vi "Acquire.vi"(8 "error in (no error)":errorcluster, 9 "Data Queue":refnum<queue>, 10 "Data Notifier":refnum<notifier>, 11 "Hardware Resources in":T1={"AI"={"task name"="", "task_ref"="", "physical channels"="Dev1/ai0:7", "channels config"={"input terminal configuration"=0, "minimum value"=-5.0, "maximum value"=5.0}, "rate"=1000.0}, "conversions"={"ai0"={"a"=0.0, "b"=0.0}, "ai1"={"a"=0.0, "b"=0.0}, "ai2"={"a"=0.0, "b"=0.0}, "ai3"={"a"=0.0, "b"=0.0}, "ai4"={"a"=0.0, "b"=0.0}}, "compteur 0"={"task name"="CTR", "task_ref"="", "ctr"="Dev1/ctr0:3", "coeff"=4000.0}, "compteur 1"={"task name"="CTR1", "task_ref"="", "ctr"="Dev1/ctr1", "coeff"=4000.0}, "compteur 2"={"task name"="CTR2", "task_ref"="", "ctr"="Dev1/ctr2", "coeff"=4000.0}, "compteur 3"={"task name"="CTR3", "task_ref"="", "ctr"="Dev1/ctr3", "coeff"=4000.0}} {"compteur 3"."coeff" format="%0.2f"; "compteur 2"."coeff" format="%0.2f"; "compteur 1"."coeff" format="%0.2f"; "compteur 0"."coeff" format="%0.2f"; "AI"."rate" format="%0.2f"; "AI"."channels config"."input terminal configuration" items=["Default"=-1, "RSE"=10083, "NRSE"=10078, "Differential"=10106, "Pseudodifferential"=12529]}) -> (0 "error out":errorcluster, 3 "Hardware Resources out":T1={"AI"={"task name"="", "task_ref"="", "physical channels"="Dev1/ai0:7", "channels config"={"input terminal configuration"=0, "minimum value"=-5.0, "maximum value"=5.0}, "rate"=1000.0}, "conversions"={"ai0"={"a"=0.0, "b"=0.0}, "ai1"={"a"=0.0, "b"=0.0}, "ai2"={"a"=0.0, "b"=0.0}, "ai3"={"a"=0.0, "b"=0.0}, "ai4"={"a"=0.0, "b"=0.0}}, "compteur 0"={"task name"="CTR", "task_ref"="", "ctr"="Dev1/ctr0:3", "coeff"=4000.0}, "compteur 1"={"task name"="CTR1", "task_ref"="", "ctr"="Dev1/ctr1", "coeff"=4000.0}, "compteur 2"={"task name"="CTR2", "task_ref"="", "ctr"="Dev1/ctr2", "coeff"=4000.0}, "compteur 3"={"task name"="CTR3", "task_ref"="", "ctr"="Dev1/ctr3", "coeff"=4000.0}} {"compteur 3"."coeff" format="%0.2f"; "compteur 2"."coeff" format="%0.2f"; "compteur 1"."coeff" format="%0.2f"; "compteur 0"."coeff" format="%0.2f"; "AI"."rate" format="%0.2f"; "AI"."channels config"."input terminal configuration" items=["Default"=-1, "RSE"=10083, "NRSE"=10078, "Differential"=10106, "Pseudodifferential"=12529]})   [LabVIEW 2014, in "PLS Acquisition.lvlib"]
doc: "Perform the acquisition. Replace the contents of this diagram with calls to acquisition hardware."
uses:
  PLS Acquisition.lvlib
  Hardware Configuration.ctl
  Settings/conversion.ctl
  <vilib>/DAQmx/read.llb/DAQmx Read (Counter DBL 1Chan 1Samp).vi
  <vilib>/DAQmx/read.llb/DAQmx Read (Analog 1D Wfm NChan NSamp).vi
  <vilib>/DAQmx/miscellaneous.llb/DAQmx Fill In Error Info.vi
  GLB_compteurs.vi
  GLB_Fsave.vi
  Settings/PLS Settings.lvlib
panel:
  out "d4":i32=10
  out "d3":i32=10
  out "d2":i32=10
  out "d1":i32=10
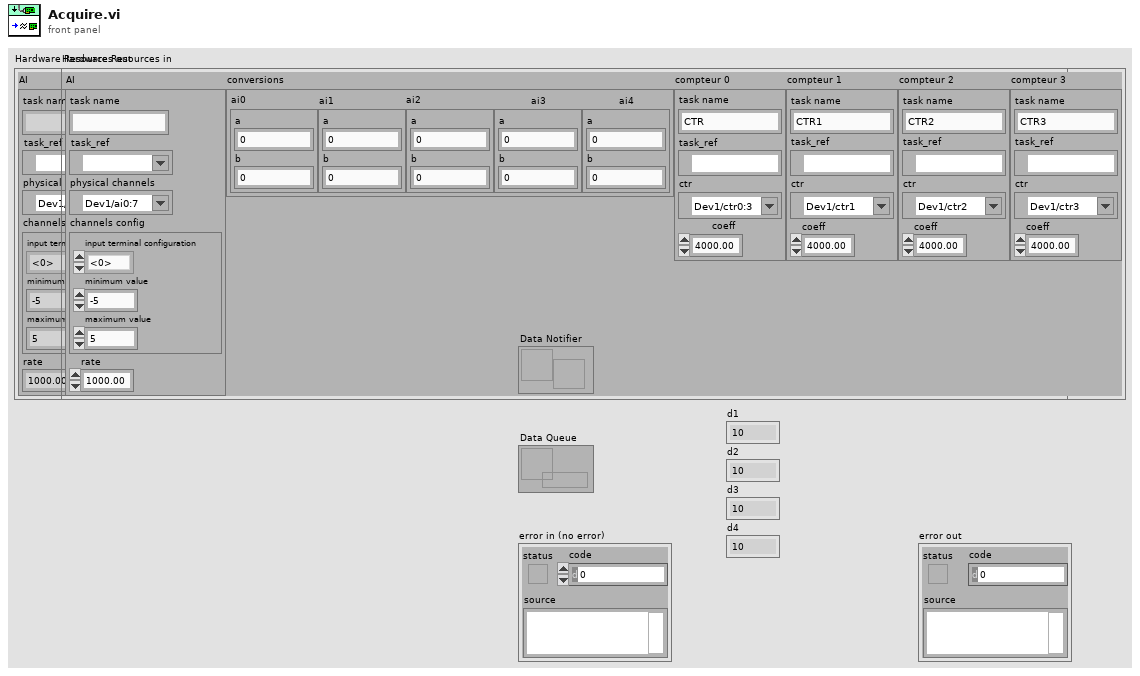
[diagram p1: front panel]
types:
  T1 = typedef "PLS Acquisition.lvlib/Hardware Configuration.ctl" = cluster{"AI":cluster{"task name":string, "task_ref":refnum<k21>, "physical channels":tag, "channels config":cluster{"input terminal configuration":i32, "minimum value":dbl, "maximum value":dbl}, "rate":dbl}, "conversions":cluster{"ai0":T2, "ai1":T2, "ai2":T2, "ai3":T2, "ai4":T2}, "compteur 0":cluster{"task name":string, "task_ref":refnum<k21>, "ctr":tag, "coeff":dbl}, "compteur 1":cluster{"task name":string, "task_ref":refnum<k21>, "ctr":tag, "coeff":dbl}, "compteur 2":cluster{"task name":string, "task_ref":refnum<k21>, "ctr":tag, "coeff":dbl}, "compteur 3":cluster{"task name":string, "task_ref":refnum<k21>, "ctr":tag, "coeff":dbl}}
  T2 = typedef "PLS Settings.lvlib/conversion.ctl" = cluster{"a":dbl, "b":dbl}
  T3 = cluster{"ai0":T2, "ai1":T2, "ai2":T2, "ai3":T2, "ai4":T2}
  T4 = cluster{"task name":string, "task_ref":refnum<k21>, "ctr":tag, "coeff":dbl}
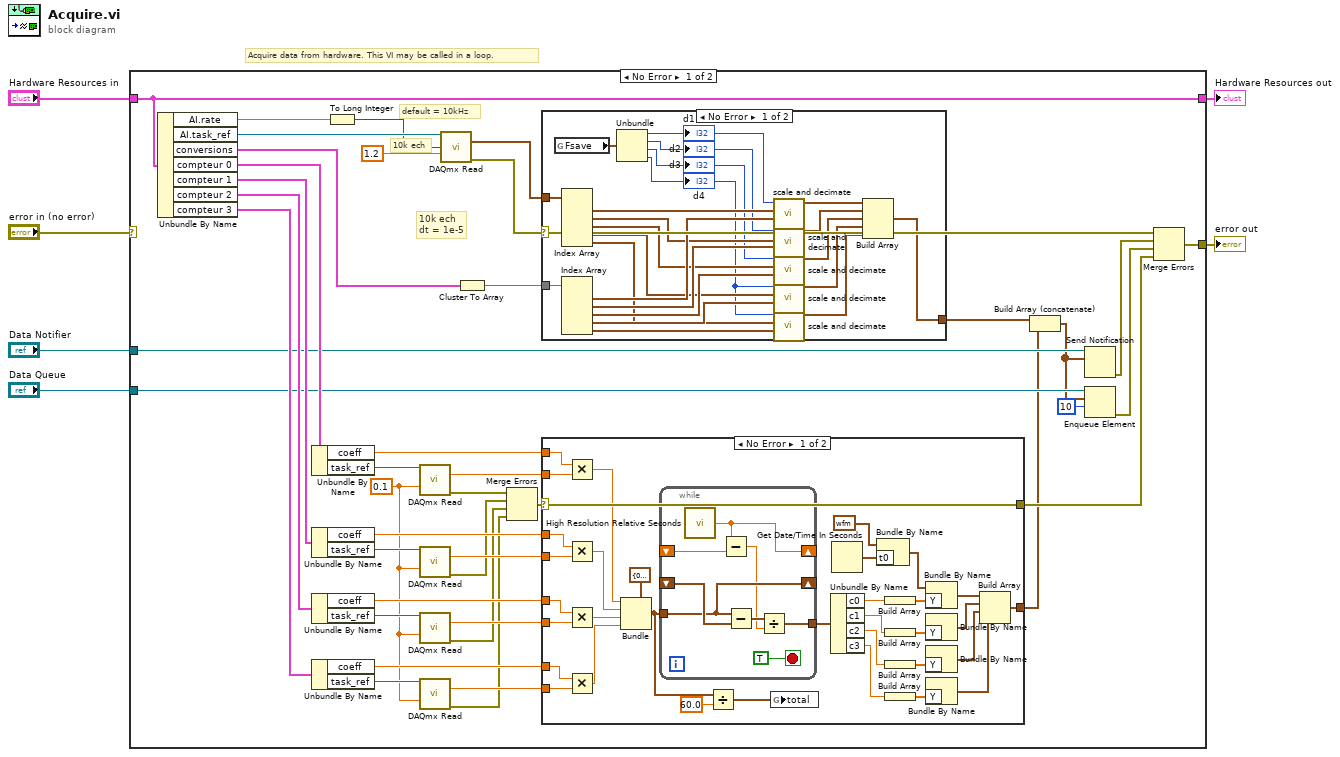
[diagram p0: block diagram]
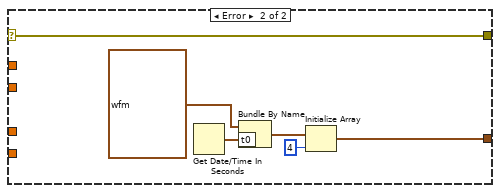
[diagram p2: hidden frame]
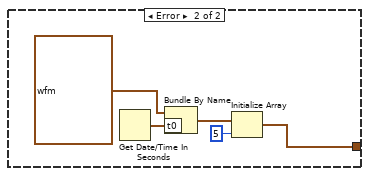
[diagram p3: hidden frame]
diagram:
  # "Acquire data from hardware. This VI may be called in a loop."
  n1 = case shown="No Error" "error in (no error)" {
    selector: "error in (no error)" -> [_ w124]
    tunnel: [w38 w124] -> w5
    tunnel: "Hardware Resources in" -> [w41 w125]
    tunnel: [w41 w125] -> w3
    tunnel: "Data Notifier" -> [w15 _]
    tunnel: "Data Queue" -> [w16 _]
    frame No Error {
      w21 = 0.1 ("timeout")
      # "10k ech\ndt = 1e-5"
      # "10k ech"
      # "default = 10kHz"
      n2 = Unbundle By Name(w41) -> ("AI.rate"=w22:dbl, "AI.task_ref"=w47:refnum<k21>, "conversions"=w43:T3, "compteur 0"=w34:T4, "compteur 1"=w29:T4, "compteur 2"=w30:T4, "compteur 3"=w31:T4)
      n3 = Unbundle By Name(w34) -> ("coeff"=w32:dbl, "task_ref"=w33:refnum<k21>)
      n4 = Unbundle By Name(w29) -> ("coeff"=w27:dbl, "task_ref"=w28:refnum<k21>)
      n5 = Unbundle By Name(w30) -> ("coeff"=w25:dbl, "task_ref"=w26:refnum<k21>)
      n6 = Unbundle By Name(w31) -> ("coeff"=w23:dbl, "task_ref"=w24:refnum<k21>)
      n7 = To Long Integer(number=w22) -> (32bit integer=w7:i32)
      n8 = call-poly <vilib>:"DAQmx Read.vi"("task/channels in"=w33, "timeout"=w21) -> ("data"=w40:dbl, "error out"=w39:errorcluster)  [unwired: 11 in, 1 out]
      n9 = call-poly <vilib>:"DAQmx Read.vi"("task/channels in"=w28, "timeout"=w21) -> ("data"=w35:dbl, "error out"=w19:errorcluster)  [unwired: 11 in, 1 out]
      n10 = call-poly <vilib>:"DAQmx Read.vi"("task/channels in"=w26, "timeout"=w21) -> ("data"=w36:dbl, "error out"=w18:errorcluster)  [unwired: 11 in, 1 out]
      n11 = call-poly <vilib>:"DAQmx Read.vi"("task/channels in"=w24, "timeout"=w21) -> ("data"=w37:dbl, "error out"=w17:errorcluster)  [unwired: 11 in, 1 out]
      n12 = call-poly <vilib>:"DAQmx Read.vi"("task/channels in"=w47, "number of samples per channel"=w7, "timeout"=1.2) -> ("data"=w45:waveform(dbl)[], "error out"=w44:errorcluster)  [unwired: 10 in, 1 out]
      n13 = Cluster To Array(cluster=w43) -> (array=w42:T2[])
      n14 = Merge Errors(w39, w19, w18, w17) -> (w20:errorcluster)
      n15 = case shown="No Error" w44 {
        tunnel: w45 -> [w118 _]
        tunnel: w42 -> [w116 _]
        tunnel: [w105 w119] -> w14
        frame No Error {
          n16 = global read "GLB_Fsave.vi" "Fsave"() -> (w100:cluster{"L1":i32, "L2":i32, "L3":i32, "L4":i32})
          n17 = Index Array(array=w118) -> (element #1=w114:waveform(dbl), element #2=w109:waveform(dbl), element #3=w108:waveform(dbl), element #4=w107:waveform(dbl), element #5=w106:waveform(dbl))  [unwired: 5 in]
          n18 = Index Array(array=w116) -> (element #1=w115:T2, element #2=w113:T2, element #3=w112:T2, element #4=w111:T2, element #5=w110:T2)  [unwired: 5 in]
          n19 = Unbundle(w100) -> ("L1"=w99:i32, "L2"=w98:i32, "L3"=w97:i32, "L4"=w96:i32)
          "d1" <- w99
          "d2" <- w98
          "d3" <- w97
          "d4" <- w96
          n20 = call "scale and decimate.vi"("scale"=w115, "Waveform in"=w114, "decimating factor"=w99) -> ("Waveform out"=w117:waveform(dbl))  [unwired: 8 in]
          n21 = call "scale and decimate.vi"("scale"=w113, "Waveform in"=w109, "decimating factor"=w98) -> ("Waveform out"=w104:waveform(dbl))  [unwired: 8 in]
          n22 = call "scale and decimate.vi"("scale"=w112, "Waveform in"=w108, "decimating factor"=w97) -> ("Waveform out"=w103:waveform(dbl))  [unwired: 8 in]
          n23 = call "scale and decimate.vi"("scale"=w111, "Waveform in"=w107, "decimating factor"=w96) -> ("Waveform out"=w102:waveform(dbl))  [unwired: 8 in]
          n24 = call "scale and decimate.vi"("scale"=w110, "Waveform in"=w106, "decimating factor"=w96) -> ("Waveform out"=w101:waveform(dbl))  [unwired: 8 in]
          n25 = Build Array(w117, w104, w103, w102, w101) -> (w105:waveform(dbl)[])
        }
        frame Error {
          n26 = Get Date/Time In Seconds() -> (seconds since 1Jan1904=w123:timestamp)
          n27 = Bundle By Name(cluster=waveform(dbl) {"t0"=timestamp(0 s since 1904-01-01), "dt"=0.1, "Y"=[nan]} ("waveform"), "t0"=w123) -> (w121:waveform(dbl))
          n28 = Initialize Array(w121, 5 ("dimension size")) -> (w119:waveform(dbl)[])
        }
      }
      n29 = case shown="No Error" w20 {
        selector: w20 -> [w80 w95]
        tunnel: w40 -> [w81 _]
        tunnel: w32 -> [w76 _]
        tunnel: [w80 w95] -> w13
        tunnel: w37 -> [w79 _]
        tunnel: w36 -> [w78 _]
        tunnel: w35 -> [w77 _]
        tunnel: w27 -> [w72 _]
        tunnel: w25 -> [w71 _]
        tunnel: w23 -> [w70 _]
        tunnel: [w51 w90] -> w8
        frame No Error {
          n30 = Multiply(x=w76, y=w81) -> (x*y=w67:dbl)
          n31 = Multiply(x=w72, y=w77) -> (x*y=w75:dbl)
          n32 = Multiply(x=w71, y=w78) -> (x*y=w74:dbl)
          n33 = Multiply(x=w70, y=w79) -> (x*y=w73:dbl)
          n34 = Bundle(cluster=cluster{"c0":dbl, "c1":dbl, "c2":dbl, "c3":dbl} {"c0"=0.0, "c1"=0.0, "c2"=0.0, "c3"=0.0} ("live"), "c0"=w67, "c1"=w75, "c2"=w74, "c3"=w73) -> (w50:cluster{"c0":dbl, "c1":dbl, "c2":dbl, "c3":dbl})
          n35 = while {
            tunnel: w50 -> [w87]
            shift-right: [w87] -> _
            shift-left: _ -> [w88]
            shift-right: [w85] -> _
            shift-left: _ -> [w84]
            tunnel: [w82] -> w69
            stop <- TRUE stop-if-true
            n36 = call <vilib>:"High Resolution Relative Seconds.vi"() -> ("relative seconds"=w85:dbl)
            n37 = Subtract(x=w85, y=w84) -> (x-y=w83:dbl)
            n38 = Subtract(x=w87, y=w88) -> (x-y=w86:cluster{"c0":dbl, "c1":dbl, "c2":dbl, "c3":dbl})
            n39 = Divide(x=w86, y=w83) -> (x/y=w82:cluster{"c0":dbl, "c1":dbl, "c2":dbl, "c3":dbl})
          }
          n40 = Divide(x=w50, y=60.0 ("timeout")) -> (x/y=w49:cluster{"c0":dbl, "c1":dbl, "c2":dbl, "c3":dbl})
          n41 = global write "GLB_compteurs.vi" "total"(w49) -> ()
          n42 = Unbundle By Name(w69) -> ("c0"=w65:dbl, "c1"=w55:dbl, "c2"=w56:dbl, "c3"=w57:dbl)
          n43 = Get Date/Time In Seconds() -> (seconds since 1Jan1904=w66:timestamp)
          n44 = Bundle By Name(cluster=waveform(dbl) {"t0"=timestamp(0 s since 1904-01-01), "dt"=0.1, "Y"=[]} ("waveform"), "t0"=w66) -> (w63:waveform(dbl))
          n45 = Build Array(w65) -> (w62:dbl[])
          n46 = Build Array(w55) -> (w60:dbl[])
          n47 = Build Array(w56) -> (w59:dbl[])
          n48 = Build Array(w57) -> (w58:dbl[])
          n49 = Bundle By Name(cluster=w63, "Y"=w62) -> (w61:waveform(dbl))
          n50 = Bundle By Name("Y"=w60) -> (w54:waveform(dbl))  [unwired: 1 in]
          n51 = Bundle By Name("Y"=w59) -> (w53:waveform(dbl))  [unwired: 1 in]
          n52 = Bundle By Name("Y"=w58) -> (w52:waveform(dbl))  [unwired: 1 in]
          n53 = Build Array(w61, w54, w53, w52) -> (w51:waveform(dbl)[])
        }
        frame Error {
          n54 = Get Date/Time In Seconds() -> (seconds since 1Jan1904=w94:timestamp)
          n55 = Bundle By Name(cluster=waveform(dbl) {"t0"=timestamp(0 s since 1904-01-01), "dt"=0.1, "Y"=[nan]} ("waveform"), "t0"=w94) -> (w92:waveform(dbl))
          n56 = Initialize Array(w92, 4 ("dimension size")) -> (w90:waveform(dbl)[])
        }
      }
      n57 = Build Array (concatenate)(w14, w8) -> (w10:waveform(dbl)[])
      n58 = Send Notification(notification=w10, notifier=w15) -> (error out=w12:errorcluster)  [unwired: 1 in, 1 out]
      n59 = Enqueue Element(queue=w16, element=w10, timeout in ms (-1)=10) -> (error out=w11:errorcluster)  [unwired: 1 in, 2 out]
      n60 = Merge Errors(w44, w12, w11, w13) -> (w38:errorcluster)
    }
    frame Error {
    }
  }
  "Hardware Resources out" <- w3
  "error out" <- w5
